vi "Notifier scenario.vi"() -> ()   [LabVIEW 2012]
panel:
  out "Process 3":i32(slide) scale=0.0..100.0
  out "Process 2":i32(slide) scale=0.0..100.0
  out "Process 1":i32(slide) scale=0.0..100.0
  out "Notification Received 3":string
  out "Notification Received 2":string
  out "Notification Received 1":string
  in  "Send Notification":bool
  in  "notification":string="instruction"
  in  "stop":bool
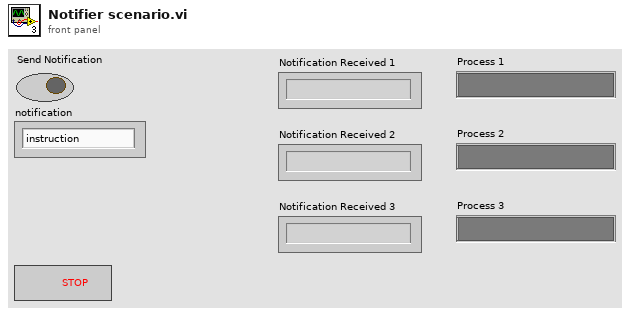
[diagram p1: front panel]
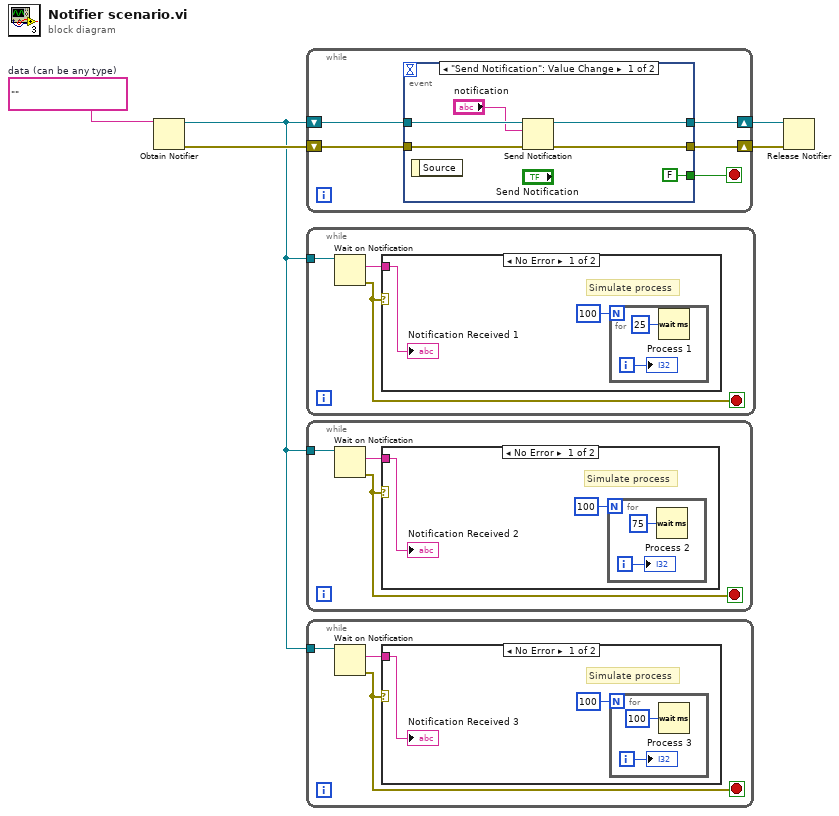
[diagram p0: block diagram]
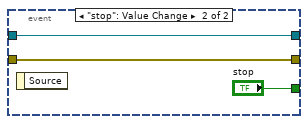
[diagram p5: hidden frame]
diagram:
  w2 = ""  # data (can be any type)
  n1 = Obtain Notifier(notification data type=w2) -> (notifier out=w1:refnum<notifier>, error out=w5:errorcluster)  [unwired: 2 in, 2 out]
  n2 = while {
    shift-right: [w9] -> w4
    shift-left: w5 -> [w8]
    shift-right: [w7] -> w3
    shift-left: w1 -> [w10]
    stop <- w6 stop-if-true
    n3 = event shown="[0] \"Send Notification\": Value Change" {
      selector: _ -> [_ _]
      dyn-events: _ -> [_ _]
      timeout: _ -> [_ _]
      tunnel: w10 -> [w16 w18]
      tunnel: [w15 w17] -> w9
      tunnel: w8 -> [w14 w17]
      tunnel: [w13 w18] -> w7
      tunnel: [FALSE ("stop") "stop"] -> w6
      event "Send Notification": Value Change {
        n4 = event-data() -> ()  [unwired: 1 in, 1 out]
        n5 = Send Notification(notification="notification", notifier=w16, error in (no error)=w14) -> (notifier out=w13:refnum<notifier>, error out=w15:errorcluster)
      }
      event "stop": Value Change {
        n6 = event-data() -> ()  [unwired: 1 in, 1 out]
      }
    }
  }
  n7 = while {
    tunnel: w1 -> [w22]
    stop <- w21 stop-if-true
    n8 = Wait on Notification(notifier=w22) -> (notification=w20:string, error out=w21:errorcluster)  [unwired: 1 in, 4 out]
    n9 = case shown="No Error" w21 {
      tunnel: w20 -> [w24 _]
      frame No Error {
        # "Simulate process"
        n10 = for {
          N: 100 -> [_]
          i -> [w26]
          n11 = Wait (ms)(milliseconds to wait=u32 25) -> ()  [unwired: 1 out]
          "Process 1" <- w26
        }
        "Notification Received 1" <- w24
      }
      frame Error {
      }
    }
  }
  n12 = while {
    tunnel: w1 -> [w29]
    stop <- w28 stop-if-true
    n13 = Wait on Notification(notifier=w29) -> (notification=w27:string, error out=w28:errorcluster)  [unwired: 1 in, 4 out]
    n14 = case shown="No Error" w28 {
      tunnel: w27 -> [w31 _]
      frame No Error {
        # "Simulate process"
        n15 = for {
          N: 100 -> [_]
          i -> [w33]
          n16 = Wait (ms)(milliseconds to wait=u32 75) -> ()  [unwired: 1 out]
          "Process 2" <- w33
        }
        "Notification Received 2" <- w31
      }
      frame Error {
      }
    }
  }
  n17 = while {
    tunnel: w1 -> [w36]
    stop <- w35 stop-if-true
    n18 = Wait on Notification(notifier=w36) -> (notification=w34:string, error out=w35:errorcluster)  [unwired: 1 in, 4 out]
    n19 = case shown="No Error" w35 {
      tunnel: w34 -> [w38 _]
      frame No Error {
        # "Simulate process"
        n20 = for {
          N: 100 -> [_]
          i -> [w40]
          n21 = Wait (ms)(milliseconds to wait=u32 100) -> ()  [unwired: 1 out]
          "Process 3" <- w40
        }
        "Notification Received 3" <- w38
      }
      frame Error {
      }
    }
  }
  n22 = Release Notifier(notifier=w3, error in (no error)=w4) -> ()  [unwired: 4 out]
